vi "negative to postive.vi"(11 "Array":dbl[](array[numeric])) -> (3 "Array 2":dbl[](array[numeric]))   [LabVIEW 2021]
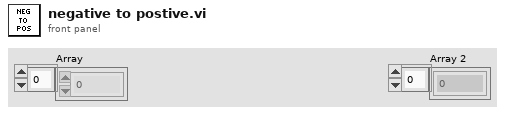
[diagram p1: front panel]
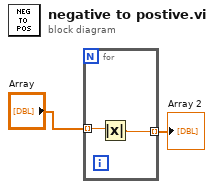
[diagram p0: block diagram]
diagram:
  n1 = for {
    tunnel: "Array" -> [w4] mode=indexing
    tunnel: [w3] -> w1 mode=indexing
    n2 = Absolute Value(x=w4) -> (abs(x)=w3:dbl)
  }
  "Array 2" <- w1
